vi "GSF_Send_Data_DAQ.vi"(8 "error in":errorcluster, 10 "AI duration (ms)":i32=1000, 11 "Digital Ports":tag="Dev1/port0") -> (0 "error out":errorcluster, 2 "data":waveform(dbl))   [LabVIEW 2021]
uses:
  <vilib>/DAQmx/write.llb/DAQmx Write (Digital 1D U32 1Chan NSamp).vi
  <vilib>/DAQmx/read.llb/DAQmx Read (Analog Wfm 1Chan NSamp).vi
  <vilib>/DAQmx/create/channels.llb/DAQmx Create Channel (DO-Digital Output).vi
  <vilib>/DAQmx/create/channels.llb/DAQmx Create Channel (CO-Pulse Generation-Ticks).vi
  <vilib>/DAQmx/configure/timing.llb/DAQmx Timing (Implicit).vi
  <vilib>/DAQmx/create/channels.llb/DAQmx Create Channel (AI-Voltage-Basic).vi
  <vilib>/DAQmx/configure/timing.llb/DAQmx Timing (Sample Clock).vi
  <vilib>/DAQmx/configure/trigger.llb/DAQmx Start Trigger (Analog Edge).vi
  Global_DAQ.vi
  <vilib>/DAQmx/create/channels.llb/DAQmx Create Channel (CO-Pulse Generation-Frequency).vi
  <vilib>/DAQmx/miscellaneous.llb/DAQmx Fill In Error Info.vi
  <vilib>/Utility/error.llb/Error Cluster From Error Code.vi
  <vilib>/ErrorRing/Error Ring.xnode
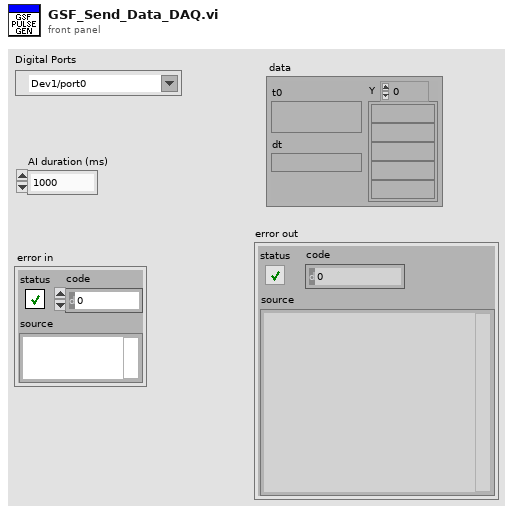
[diagram p1: front panel]
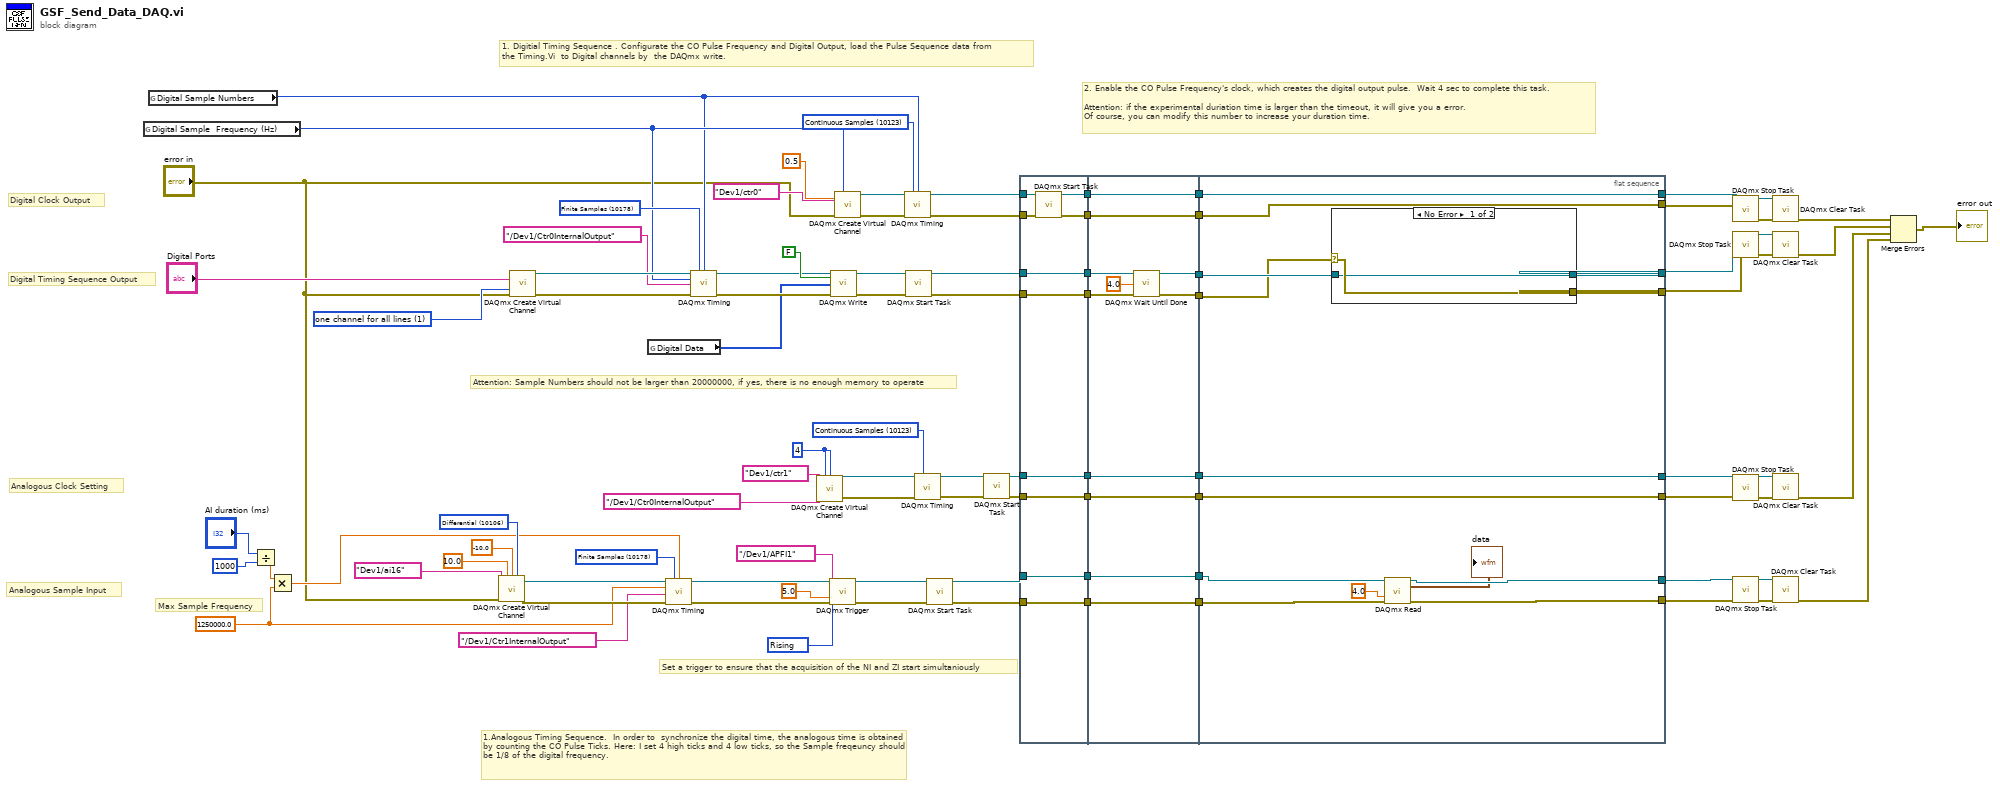
[diagram p0: block diagram]
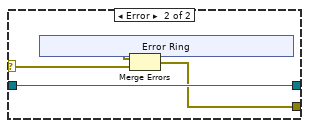
[diagram p2: hidden frame]
diagram:
  w34 = 1250000.0 ("rate")
  w37 = 10106 items=["Default"=-1, "RSE"=10083, "NRSE"=10078, "Differential"=10106, "Pseudodifferential"=12529] ("input terminal configuration")
  w39 = 10280 items=["Rising"=10280, "Falling"=10171] ("slope")
  w40 = 10178 items=["Finite Samples"=10178, "Continuous Samples"=10123, "Hardware Timed Single Point"=12522] ("sample mode")
  w54 = 10123 items=["Finite Samples"=10178, "Continuous Samples"=10123, "Hardware Timed Single Point"=12522] ("sample mode")
  w55 = u32 4 ("low ticks")
  w83 = 10178 items=["Finite Samples"=10178, "Continuous Samples"=10123, "Hardware Timed Single Point"=12522] ("sample mode")
  w84 = 1 items=["one channel for each line", "one channel for all lines"] ("line grouping")
  w89 = 10123 items=["Finite Samples"=10178, "Continuous Samples"=10123, "Hardware Timed Single Point"=12522] ("sample mode")
  # "Analogous Sample Input"
  # "Analogous Clock Setting"
  # "Digital Timing Sequence Output"
  # "Digital Clock Output"
  # "Set a trigger to ensure that the acquisition of the NI and ZI start simultaniously"
  # "1.Analogous Timing Sequence.  In order to  synchronize the digital time, the analogous time is obtained by counting the CO Pulse Ticks. Here: I set 4 high ticks and 4 low ticks, so the Sample freqeuncy should be 1/8 of the digital frequency."
  # "Max Sample Frequency"
  # "Attention: Sample Numbers should not be larger than 20000000, if yes, there is no enough memory to operate"
  # "2. Enable the CO Pulse Frequency's clock, which creates the digital output pulse.  Wait 4 sec to complete this task.    \n\nAttention: if the experimental duriation time is larger than the timeout, it will give you a error.\nOf course, you can modify this number to increase your duration time."
  # "1. Digitial Timing Sequence . Configurate the CO Pulse Frequency and Digital Output, load the Pulse Sequence data from\nthe Timing.Vi  to Digital channels by  the DAQmx write."
  n1 = global read "Global_DAQ.vi" "Digital Sample  Frequency (Hz)"() -> (w66:u32)
  n2 = global read "Global_DAQ.vi" "Digital Sample Numbers"() -> (w63:u32)
  n3 = Divide(x="AI duration (ms)", y=1000) -> (x/y=w35:dbl)
  n4 = Multiply(x=w35, y=w34) -> (x*y=w32:dbl)
  n5 = call-poly <vilib>:"DAQmx Create Virtual Channel.vi"("maximum value"=10.0, "minimum value"=-10.0, "input terminal configuration"=w37, "physical channels"=tag "Dev1/ai16", "error in"="error in") -> ("task out"=w48:refnum<k21>, "error out"=w47:errorcluster)  [unwired: 9 in]
  n6 = call-poly <vilib>:"DAQmx Create Virtual Channel.vi"("lines"="Digital Ports", "line grouping"=w84, "error in"="error in") -> ("task out"=w88:refnum<k21>, "error out"=w87:errorcluster)  [unwired: 11 in]
  n7 = global read "Global_DAQ.vi" "Digital Data"() -> (w60:u32[])
  n8 = call-poly <vilib>:"DAQmx Timing.vi"("task/channels in"=w48, "sample mode"=w40, "samples per channel"=w32, "rate"=w34, "source"=tag "/Dev1/Ctr1InternalOutput", "error in"=w47) -> ("task out"=w45:refnum<k21>, "error out"=w44:errorcluster)  [unwired: 8 in]
  n9 = call-poly <vilib>:"DAQmx Timing.vi"("task/channels in"=w88, "sample mode"=w83, "samples per channel"=w63, "rate"=w66, "source"=tag "/Dev1/Ctr0InternalOutput", "error in"=w87) -> ("task out"=w62:refnum<k21>, "error out"=w61:errorcluster)  [unwired: 8 in]
  n10 = call-poly <vilib>:"DAQmx Create Virtual Channel.vi"("high ticks"=w55, "low ticks"=w55, "counter"=tag "Dev1/ctr1", "source of ticks"=tag "/Dev1/Ctr0InternalOutput") -> ("task out"=w57:refnum<k21>, "error out"=w56:errorcluster)  [unwired: 10 in]
  n11 = call-poly <vilib>:"DAQmx Trigger.vi"("task/channels in"=w45, "source"=tag "/Dev1/APFI1", "slope"=w39, "level"=5.0, "error in"=w44) -> ("task out"=w42:refnum<k21>, "error out"=w41:errorcluster)  [unwired: 9 in]
  n12 = call-poly <vilib>:"DAQmx Write.vi"("task/channels in"=w62, "auto start"=FALSE, "data"=w60, "error in"=w61) -> ("task out"=w80:refnum<k21>, "error out"=w79:errorcluster)  [unwired: 9 in, 1 out]
  n13 = call-poly <vilib>:"DAQmx Create Virtual Channel.vi"("frequency"=w66, "duty cycle"=0.5, "counter"=tag "Dev1/ctr0", "error in"="error in") -> ("task out"=w81:refnum<k21>, "error out"=w90:errorcluster)  [unwired: 10 in]
  n14 = call-poly <vilib>:"DAQmx Timing.vi"("task/channels in"=w81, "sample mode"=w89, "samples per channel"=w63, "error in"=w90) -> ("task out"=w85:refnum<k21>, "error out"=w64:errorcluster)  [unwired: 10 in]
  n15 = call <vilib>:"DAQmx Start Task.vi"("task/channels in"=w80, "error in"=w79) -> ("task out"=w78:refnum<k21>, "error out"=w65:errorcluster)  [unwired: 12 in]
  n16 = call-poly <vilib>:"DAQmx Timing.vi"("task/channels in"=w57, "sample mode"=w54, "error in"=w56) -> ("task out"=w53:refnum<k21>, "error out"=w52:errorcluster)  [unwired: 11 in]
  n17 = call <vilib>:"DAQmx Start Task.vi"("task/channels in"=w42, "error in"=w41) -> ("task out"=w31:refnum<k21>, "error out"=w30:errorcluster)  [unwired: 12 in]
  n18 = call <vilib>:"DAQmx Start Task.vi"("task/channels in"=w53, "error in"=w52) -> ("task out"=w29:refnum<k21>, "error out"=w28:errorcluster)  [unwired: 12 in]
  n19 = flat-sequence {
    tunnel: [w101] -> w27
    tunnel: [w100] -> w25
    tunnel: [w99] -> w23
    tunnel: [w98] -> w21
    tunnel: w85 -> [w103]
    tunnel: w64 -> [w102]
    tunnel: w78 -> [w99]
    tunnel: w65 -> [w98]
    tunnel: w31 -> [w95]
    tunnel: w30 -> [w94]
    tunnel: w29 -> [w97]
    tunnel: w28 -> [w96]
    tunnel: [w97] -> w19
    tunnel: [w96] -> w17
    tunnel: [w95] -> w15
    tunnel: [w94] -> w13
    tunnel: w27 -> [w114]
    tunnel: [w114] -> w26
    tunnel: w25 -> [w113]
    tunnel: [w113] -> w24
    tunnel: w23 -> [w108]
    tunnel: [w106] -> w22
    tunnel: w21 -> [w107]
    tunnel: [w105] -> w20
    tunnel: w19 -> [w112]
    tunnel: [w112] -> w18
    tunnel: w17 -> [w111]
    tunnel: [w111] -> w16
    tunnel: w15 -> [w110]
    tunnel: [w110] -> w14
    tunnel: w13 -> [w109]
    tunnel: [w109] -> w12
    tunnel: w26 -> [w128]
    tunnel: w24 -> [w124]
    tunnel: w22 -> [w126]
    tunnel: w20 -> [w123]
    tunnel: [w128] -> w73
    tunnel: [w127] -> w70
    tunnel: [w125] -> w72
    tunnel: [w124] -> w71
    tunnel: w18 -> [w116]
    tunnel: w16 -> [w117]
    tunnel: w14 -> [w120]
    tunnel: w12 -> [w121]
    tunnel: [w119] -> w7
    tunnel: [w118] -> w6
    tunnel: [w117] -> w5
    tunnel: [w116] -> w4
    frame #0 {
      n20 = call <vilib>:"DAQmx Start Task.vi"("task/channels in"=w103, "error in"=w102) -> ("task out"=w101:refnum<k21>, "error out"=w100:errorcluster)  [unwired: 12 in]
    }
    frame #1 {
      n21 = call <vilib>:"DAQmx Wait Until Done.vi"("task/channels in"=w108, "timeout (sec)"=4.0, "error in"=w107) -> ("task out"=w106:refnum<k21>, "error out"=w105:errorcluster)  [unwired: 11 in]
    }
    frame #2 {
      n22 = case shown="No Error" w123 {
        selector: w123 -> [w130 w132]
        tunnel: [w130 w131] -> w127
        tunnel: w126 -> [w129 w134]
        tunnel: [w129 w134] -> w125
        frame No Error {
        }
        frame Error {
          n23 = xnode "Error Ring"() -> ("error out"=w133:errorcluster)
          n24 = Merge Errors(w133, w132) -> (w131:errorcluster)
        }
      }
      n25 = call-poly <vilib>:"DAQmx Read.vi"("task/channels in"=w120, "timeout"=4.0, "error in"=w121) -> ("task out"=w118:refnum<k21>, "data"=→"data":waveform(dbl), "error out"=w119:errorcluster)  [unwired: 10 in]
    }
  }
  n26 = call <vilib>:"DAQmx Stop Task.vi"("task/channels in"=w73, "error in"=w71) -> ("task out"=w75:refnum<k21>, "error out"=w74:errorcluster)  [unwired: 12 in]
  n27 = call <vilib>:"DAQmx Stop Task.vi"("task/channels in"=w72, "error in"=w70) -> ("task out"=w77:refnum<k21>, "error out"=w76:errorcluster)  [unwired: 12 in]
  n28 = call <vilib>:"DAQmx Stop Task.vi"("task/channels in"=w4, "error in"=w5) -> ("task out"=w11:refnum<k21>, "error out"=w10:errorcluster)  [unwired: 12 in]
  n29 = call <vilib>:"DAQmx Stop Task.vi"("task/channels in"=w6, "error in"=w7) -> ("task out"=w9:refnum<k21>, "error out"=w8:errorcluster)  [unwired: 12 in]
  n30 = call <vilib>:"DAQmx Clear Task.vi"("task in"=w75, "error in"=w74) -> ("error out"=w69:errorcluster)  [unwired: 13 in]
  n31 = call <vilib>:"DAQmx Clear Task.vi"("task in"=w77, "error in"=w76) -> ("error out"=w68:errorcluster)  [unwired: 13 in]
  n32 = call <vilib>:"DAQmx Clear Task.vi"("task in"=w11, "error in"=w10) -> ("error out"=w3:errorcluster)  [unwired: 13 in]
  n33 = call <vilib>:"DAQmx Clear Task.vi"("task in"=w9, "error in"=w8) -> ("error out"=w2:errorcluster)  [unwired: 13 in]
  n34 = Merge Errors(w69, w68, w3, w2) -> (→"error out":errorcluster)
